vi "SetupFifo.vi"(7 "file path (use dialog)":path, 8 "Force Num Array":i32, 9 "MaxNumFileWrite":i32=255, 10 "Fifo Time Out":i32=500, 11 "Fifo Size":u32=8192) -> (3 "Data Logging Param":T1)   [LabVIEW 2016, in "kevLib2011.lvlib"]
uses:
  kevLib2011.lvlib
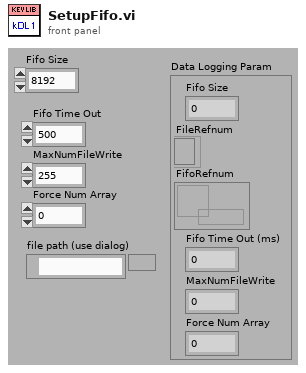
[diagram p1: front panel]
types:
  T1 = cluster{"Fifo Size":u32, "FileRefnum":refnum<file>, "FifoRefnum":refnum<k33>, "Fifo Time Out (ms)":i32, "MaxNumFileWrite":i32, "Force Num Array":i32}
  T2 = enum16{"open", "replace", "create", "open or create", "replace or create", "replace or create with confirmation"}
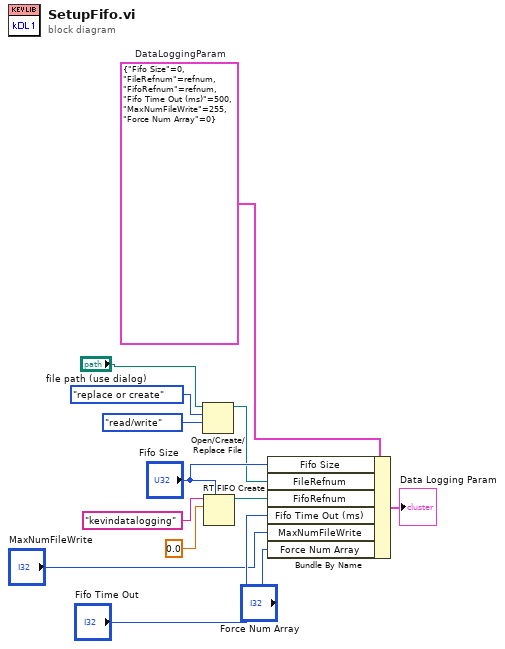
[diagram p0: block diagram]
diagram:
  w9 = T1 {"Fifo Size"=0, "FileRefnum"=refnum, "FifoRefnum"=refnum, "Fifo Time Out (ms)"=500, "MaxNumFileWrite"=255, "Force Num Array"=0}  # DataLoggingParam
  n1 = Open/Create/Replace File(file path (use dialog)="file path (use dialog)", operation (0:open)=T2."replace or create", access (0:read/write)=enum16{"read/write", "read-only", "write-only"}."read/write") -> (refnum out=w7:refnum<file>)  [unwired: 3 in, 2 out]
  n2 = RT FIFO Create(0:"kevindatalogging" ("name (unnamed)"), 1:0.0, 4:"Fifo Size") -> (8:w6:refnum<k33>)  [unwired: 5 in, 2 out]
  n3 = Bundle By Name(cluster=w9, "Fifo Size"="Fifo Size", "FileRefnum"=w7, "FifoRefnum"=w6, "Fifo Time Out (ms)"="Fifo Time Out", "MaxNumFileWrite"="MaxNumFileWrite", "Force Num Array"="Force Num Array") -> (→"Data Logging Param":T1)
